vi "TurretOffsetCoordinateTransform.vi"(8 "Robot_Heading_(deg)":dbl, 9 "Turret_Y_Offset_(in)":dbl, 10 "Turret_X_Offset_(in)":dbl) -> (1 "Turret_Delta_Y":dbl, 2 "Turret_Delta_X":dbl)   [LabVIEW 2019]
uses:
  constants.vi
  sensors.vi
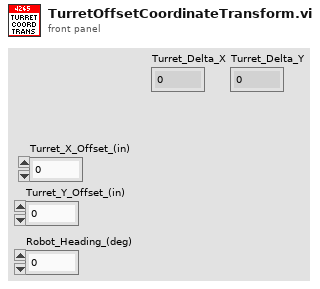
[diagram p1: front panel]
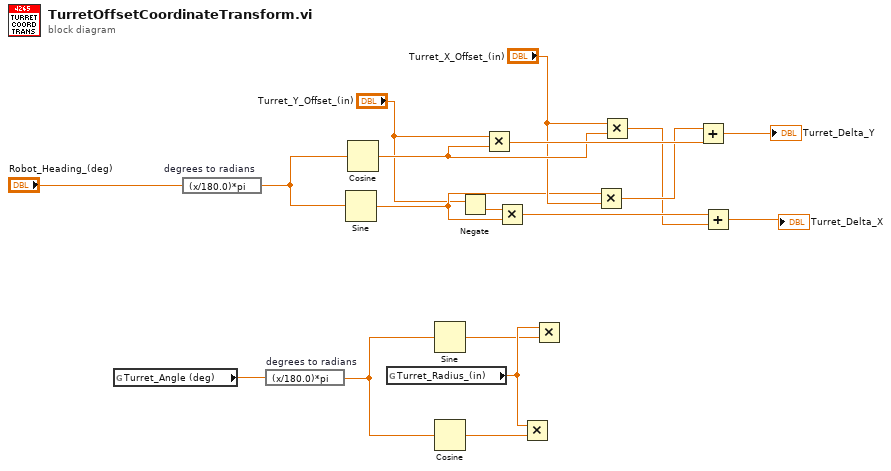
[diagram p0: block diagram]
diagram:
  n1 = global read "sensors.vi" "Turret_Angle (deg)"() -> (w16:dbl)
  n2 = expression code="(x/180.0)*pi" "degrees to radians"("Robot_Heading_(deg)") -> (w17:dbl)
  n3 = expression code="(x/180.0)*pi" "degrees to radians"(w16) -> (w15:dbl)
  n4 = Sine(x=w17) -> (sin(x)=w5:dbl)
  n5 = Cosine(x=w17) -> (cos(x)=w9:dbl)
  n6 = global read "constants.vi" "Turret_Radius_(in)"() -> (w13:dbl)
  n7 = Sine(x=w15) -> (sin(x)=w12:dbl)
  n8 = Cosine(x=w15) -> (cos(x)=w14:dbl)
  n9 = Negate(x="Turret_Y_Offset_(in)") -> (-x=w1:dbl)
  n10 = Multiply(x="Turret_Y_Offset_(in)", y=w9) -> (x*y=w11:dbl)
  n11 = Multiply(x=w1, y=w5) -> (x*y=w8:dbl)
  n12 = Multiply(x=w13, y=w14) -> ()  [unwired: 1 out]
  n13 = Multiply(x=w13, y=w12) -> ()  [unwired: 1 out]
  n14 = Multiply(x=w5, y="Turret_X_Offset_(in)") -> (x*y=w10:dbl)
  n15 = Multiply(x="Turret_X_Offset_(in)", y=w9) -> (x*y=w7:dbl)
  n16 = Add(x=w10, y=w11) -> (x+y=→"Turret_Delta_Y":dbl)
  n17 = Add(x=w8, y=w7) -> (x+y=→"Turret_Delta_X":dbl)
